vi "Read Analog and Build Waveform.vi"(0 "LINX Resource in":T1, 1 "Analog Channel":u8, 5 "Sampling Duration (s)":dbl, 7 "Sampling Frequency (Hz)":dbl, 11 "Error In":errorcluster) -> (4 "LINX Resource out":T1, 6 "mean dt":dbl, 8 "STD dt":dbl, 10 "Raw Voltage":dbl, 14 "Raw Signal Waveform Out":waveform(dbl), 15 "Error Out":errorcluster)   [LabVIEW 2025]
uses:
  <vilib>/MakerHub/LINX/Private/Type Defs/LINX Ref.ctl
  <vilib>/MakerHub/LINX/Private/Type Defs/Platform.ctl
  <vilib>/MakerHub/LINX/Private/Type Defs/Interface.ctl
  <vilib>/MakerHub/LINX/Private/Device/Type Defs/LINX Device Config.ctl
  <vilib>/MakerHub/LINX/Private/Device/Type Defs/TCP Config.ctl
  <vilib>/MakerHub/LINX/Private/Device/Type Defs/Channels.ctl
  <vilib>/MakerHub/LINX/Public/Peripherals/Analog/Analog Read 1 Chan.vi
  <vilib>/MakerHub/LINX/Public/Peripherals/Analog/Analog Read N Chans.vi
  <vilib>/MakerHub/LINX/Private/Local IO/LinxAnalogRead.vi
  <vilib>/MakerHub/LINX/Public/Utilities/Check Channel.vi
  <vilib>/MakerHub/LINX/Private/Utilties/Generate Error.vi
  <vilib>/MakerHub/LINX/LMH-LINX.lvlib
  <vilib>/Analysis/NI_AALBase.lvlib
  <vilib>/MakerHub/LINX/Private/Device/Device.lvlib
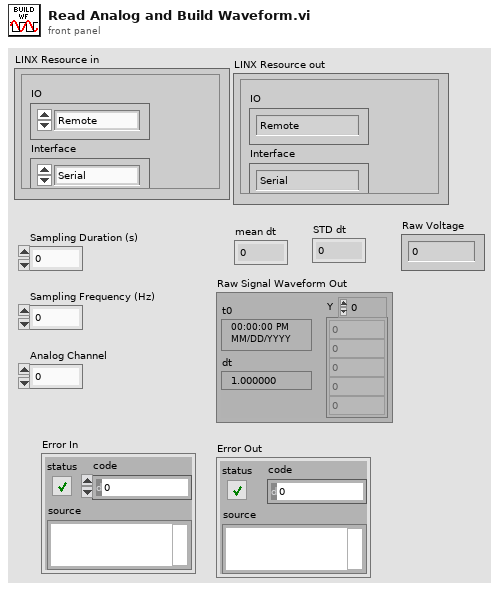
[diagram p1: front panel]
types:
  T1 = typedef "LMH-LINX.lvlib/LINX Ref.ctl" = cluster{"IO":T2, "Interface":T3, "LINX Device Config":T4}
  T2 = typedef "LMH-LINX.lvlib/Platform.ctl" = enum16{"Remote", "Local"}
  T3 = typedef "LMH-LINX.lvlib/Interface.ctl" = enum16{"Serial", "TCP"}
  T4 = typedef "LMH-LINX.lvlib/Device.lvlib/LINX Device Config.ctl" = cluster{"Interface":T3, "COM Port":refnum<visa-resource-name>, "TCP Configuration":T5, "Device Family":u8, "Device ID":u8, "Device Name":string, "TCP Ref":refnum<k5>, "Channels":T6}
  T5 = typedef "LMH-LINX.lvlib/Device.lvlib/TCP Config.ctl" = cluster{"IP Address":string, "Port":u16}
  T6 = typedef "LMH-LINX.lvlib/Channels.ctl" = cluster{"DI":u8[], "DO":u8[], "AI":u8[], "AO":u8[], "PWM":u8[], "QE":u8[], "UART":u8[], "I2C 2":u8[], "SPI":u8[], "CAN":u8[], "Servo":u8[], "AI Ref (V)":dbl, "AI Resolution (Bits)":u8, "AO Ref (V)":dbl, "AO Resolution (Bits)":u8}
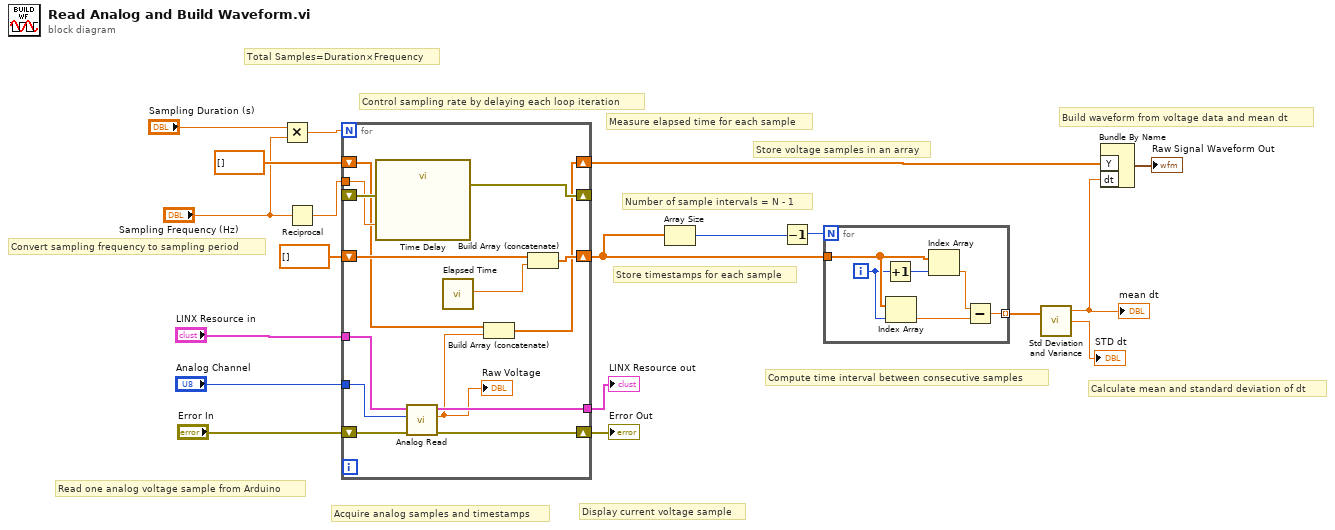
[diagram p0: block diagram]
diagram:
  # "Measure elapsed time for each sample"
  # "Build waveform from voltage data and mean dt"
  # "Calculate mean and standard deviation of dt"
  # "Compute time interval between consecutive samples"
  # "Number of sample intervals = N - 1"
  # "Store timestamps for each sample"
  # "Store voltage samples in an array"
  # "Display current voltage sample"
  # "Read one analog voltage sample from Arduino"
  # "Acquire analog samples and timestamps"
  # "Control sampling rate by delaying each loop iteration"
  # "Convert sampling frequency to sampling period"
  # "Total Samples=Duration×Frequency"
  n1 = Multiply(x="Sampling Duration (s)", y="Sampling Frequency (Hz)") -> (x*y=w8:dbl)
  n2 = Reciprocal(x="Sampling Frequency (Hz)") -> (1/x=w4:dbl)
  n3 = for {
    N: w8 -> [_]
    tunnel: "LINX Resource in" -> [w27]
    shift-right: [w32] -> _
    shift-left: _ -> [w33]
    tunnel: "Analog Channel" -> [w23]
    tunnel: w4 -> [w31]
    shift-right: [w28] -> w11
    shift-left: dbl[] [] -> [w29]
    tunnel: [w25] -> w9
    shift-right: [w22] -> w17
    shift-left: dbl[] [] -> [w21]
    shift-right: [w24] -> w10
    shift-left: "Error In" -> [w26]
    n4 = call "Time Delay"("error in (no error)"=w33, "Delay Time (s)"=w31) -> ("error out"=w32:errorcluster)  [unwired: 9 in]
    n5 = call-poly <vilib>:"Analog Read.vi"("Error In"=w26, "Analog Channel"=w23, "LINX Resource"=w27) -> ("Error Out"=w24:errorcluster, "Voltage"=w20:dbl, "LINX Resource"=w25:T1)  [unwired: 5 in, 1 out]
    "Raw Voltage" <- w20
    n6 = call "Elapsed Time"() -> ("Elapsed Time (s)"=w30:dbl)  [unwired: 12 in, 7 out]
    n7 = Build Array (concatenate)(w21, w20) -> (w22:dbl[])
    n8 = Build Array (concatenate)(w29, w30) -> (w28:dbl[])
  }
  "Error Out" <- w10
  "LINX Resource out" <- w9
  n9 = Array Size(array=w11) -> (size(s)=w12:i32)
  n10 = Decrement(x=w12) -> (x-1=w13:i32)
  n11 = for {
    N: w13 -> [_]
    tunnel: w11 -> [w39]
    tunnel: [w34] -> w15 mode=indexing
    i -> [w37]
    n12 = Increment(x=w37) -> (x+1=w38:i32)
    n13 = Index Array(array=w39, index=w37) -> (element=w35:dbl)
    n14 = Index Array(array=w39, index=w38) -> (element=w36:dbl)
    n15 = Subtract(x=w36, y=w35) -> (x-y=w34:dbl)
  }
  n16 = call <vilib>:"Std Deviation and Variance.vi"("X"=w15) -> ("mean"=w19:dbl, "standard deviation"=→"STD dt":dbl)  [unwired: 1 in, 1 out]
  "mean dt" <- w19
  n17 = Bundle By Name("Y"=w17, "dt"=w19) -> (→"Raw Signal Waveform Out":waveform(dbl))  [unwired: 1 in]
